vi "Chart_Formula_Manual_Fill.vi"(8 "error in (no error)":errorcluster, 10 "Max Voltage":dbl, 11 "Min Voltage":dbl) -> ()   [LabVIEW 2020]
uses:
  Global 1.vi
panel:
  out "Chosen Max Voltage":dbl
  out "Chosen Min Voltage":dbl
  out "Dummy Array":dbl[](array[numeric])
  out "size(s)":i32
  out "Output Array":dbl[](array[numeric])
  out "error out":errorcluster
  in  "Confirm Filled-up Test Voltages  ?":bool
  in  "Manual Fill In":dbl[](array[numeric])
  # "NOTE ON THE CHOSEN MIN & MAX VOLTAGE :"
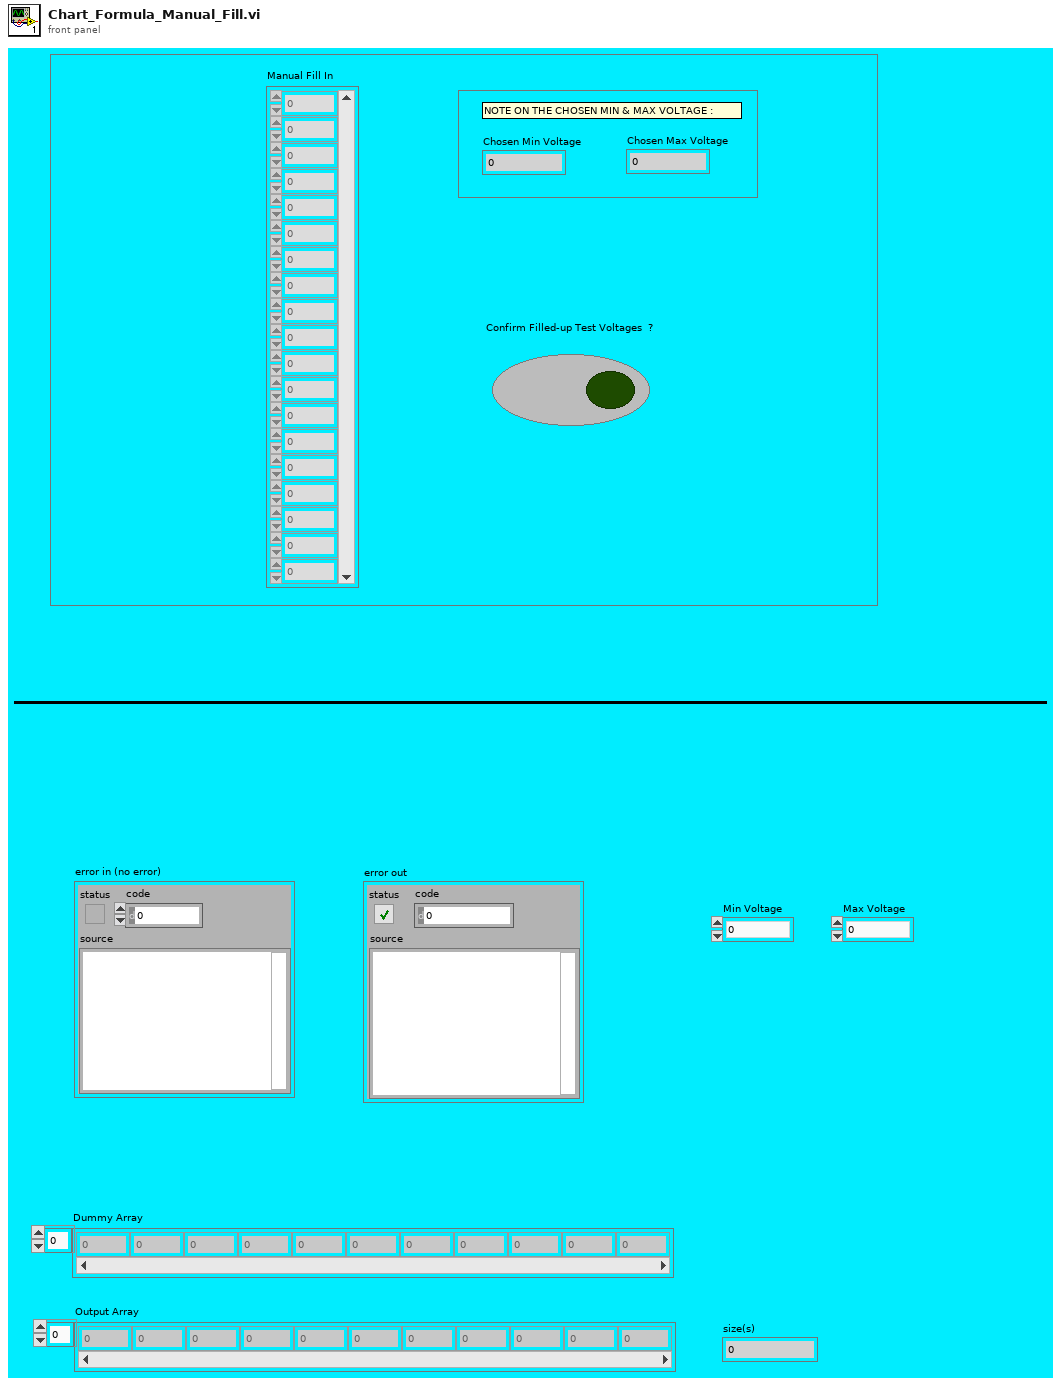
[diagram p1: front panel]
types:
  T1 = enum32{"Invalid", "Standard", "Closed", "Hidden", "Minimized", "Maximized"}
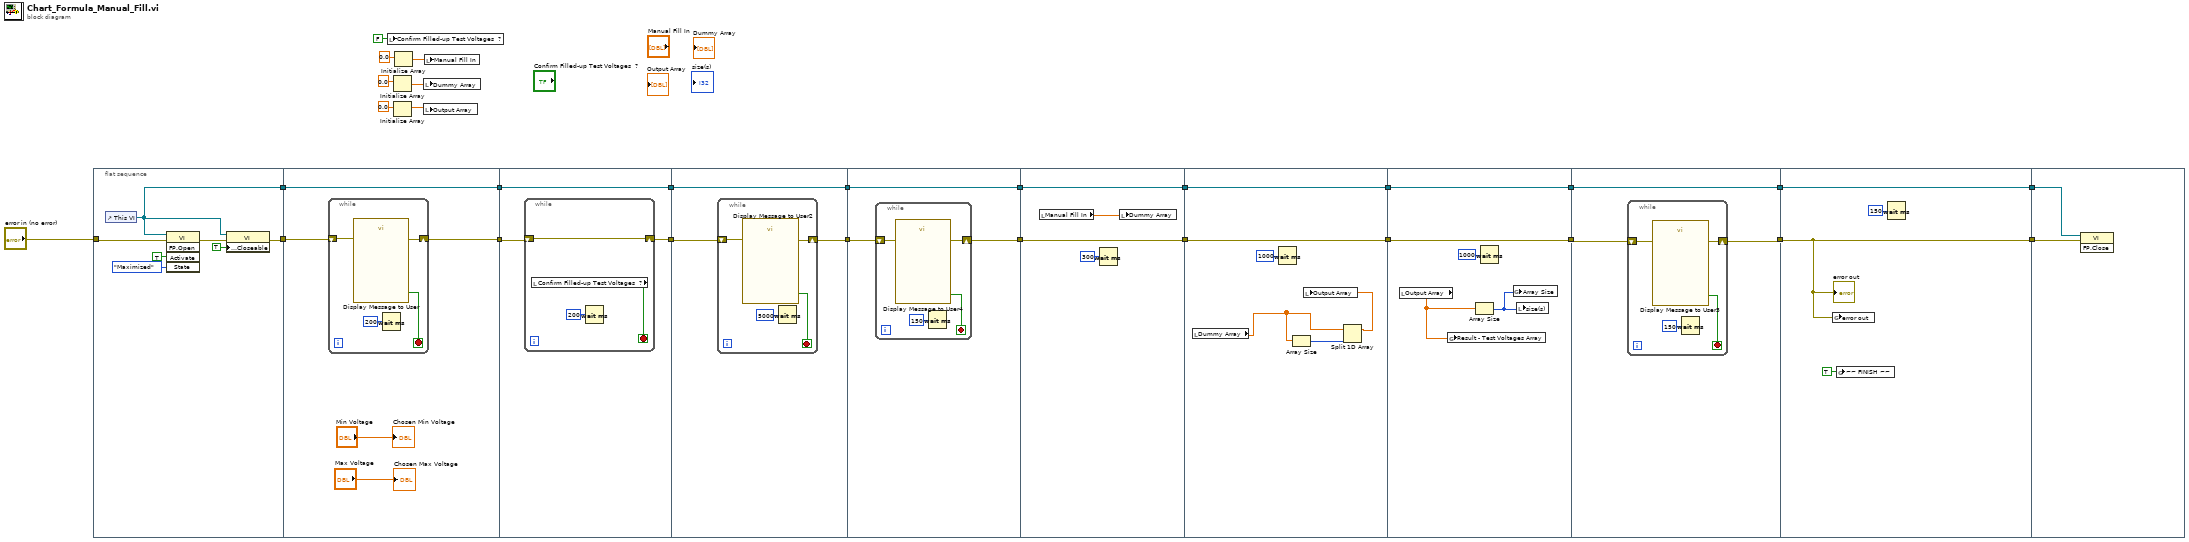
[diagram p0: block diagram]
diagram:
  n1 = flat-sequence {
    tunnel: "error in (no error)" -> [w33]
    tunnel: [w30] -> w23
    tunnel: [w29] -> w19
    tunnel: [w39] -> w25
    tunnel: w23 -> [w40]
    tunnel: [w38] -> w20
    tunnel: w19 -> [w38]
    tunnel: w25 -> [w47]
    tunnel: [w46] -> w22
    tunnel: [w45] -> w21
    tunnel: w20 -> [w45]
    tunnel: w22 -> [w53]
    tunnel: [w52] -> w6
    tunnel: w21 -> [w51]
    tunnel: [w51] -> w4
    tunnel: w6 -> [w59]
    tunnel: [w58] -> w5
    tunnel: w4 -> [w60]
    tunnel: [w60] -> w3
    tunnel: w5 -> [w68]
    tunnel: [w68] -> w18
    tunnel: [w67] -> w17
    tunnel: w3 -> [w67]
    tunnel: w18 -> [w74]
    tunnel: [w74] -> w12
    tunnel: w17 -> [w73]
    tunnel: [w73] -> w11
    tunnel: w12 -> [w79]
    tunnel: [w79] -> w10
    tunnel: w11 -> [w78]
    tunnel: [w78] -> w8
    tunnel: w10 -> [w81]
    tunnel: [w80] -> w9
    tunnel: w8 -> [w82]
    tunnel: [w82] -> w7
    tunnel: w9 -> [w88]
    tunnel: w7 -> [w89]
    tunnel: [w89] -> w2
    tunnel: [w88] -> w1
    tunnel: w2 -> [w92]
    tunnel: w1 -> [w91]
    frame #0 {
      n2 = control-ref of="This VI"() -> (w29:refnum<vi>)
      n3 = invoke class="VI" method="FP.Open"(reference=w29, error in=w33, "Activate"=TRUE ("Activate?"), "State"=T1."Maximized") -> (error out=w31:errorcluster)  [unwired: 1 in, 4 out]
      n4 = property class="VI"(reference=w29, error in=w31, "Front Panel.Closeable"=TRUE ("Front Panel Window:Closeable")) -> (error out=w30:errorcluster)  [unwired: 1 out]
    }
    frame #1 {
      n5 = while {
        shift-right: [w43] -> w39
        shift-left: w40 -> [w44]
        stop <- w41 stop-if-true
        n6 = call "Display Message to User"("error in (no error)"=w44) -> ("error out"=w43:errorcluster, "OK"=w41:bool)  [unwired: 9 in]
        n7 = Wait (ms)(milliseconds to wait=u32 200) -> ()  [unwired: 1 out]
      }
      "Chosen Min Voltage" <- "Min Voltage"
      "Chosen Max Voltage" <- "Max Voltage"
    }
    frame #2 {
      n8 = while {
        shift-right: [w49] -> w46
        shift-left: w47 -> [w49]
        stop <- w48 stop-if-true
        n9 = local read "Confirm Filled-up Test Voltages  ?"() -> (w48:bool)
        n10 = Wait (ms)(milliseconds to wait=u32 200) -> ()  [unwired: 1 out]
      }
    }
    frame #3 {
      n11 = while {
        shift-right: [w56] -> w52
        shift-left: w53 -> [w57]
        stop <- w54 stop-if-true
        n12 = call "Display Message to User2"("error in (no error)"=w57) -> ("error out"=w56:errorcluster, "YES"=w54:bool)  [unwired: 9 in]
        n13 = Wait (ms)(milliseconds to wait=u32 5000) -> ()  [unwired: 1 out]
      }
    }
    frame #4 {
      n14 = while {
        shift-right: [w63] -> w58
        shift-left: w59 -> [w64]
        stop <- w62 stop-if-true
        n15 = call "Display Message to User4"("error in (no error)"=w64) -> ("error out"=w63:errorcluster, "OK"=w62:bool)  [unwired: 9 in]
        n16 = Wait (ms)(milliseconds to wait=u32 150) -> ()  [unwired: 1 out]
      }
    }
    frame #5 {
      n17 = local read "Manual Fill In"() -> (w66:dbl[])
      n18 = Wait (ms)(milliseconds to wait=u32 300) -> ()  [unwired: 1 out]
      n19 = local write "Dummy Array"(w66) -> ()
    }
    frame #6 {
      n20 = local read "Dummy Array"() -> (w70:dbl[])
      n21 = Wait (ms)(milliseconds to wait=u32 1000) -> ()  [unwired: 1 out]
      n22 = Array Size(array=w70) -> (size(s)=w69:i32)
      n23 = Split 1D Array(array=w70, index=w69) -> (first subarray=w71:dbl[])  [unwired: 1 out]
      n24 = local write "Output Array"(w71) -> ()
    }
    frame #7 {
      n25 = local read "Output Array"() -> (w76:dbl[])
      n26 = global write "Global 1.vi" "Result - Test Voltages Array"(w76) -> ()
      n27 = Array Size(array=w76) -> (size(s)=w77:i32)
      n28 = Wait (ms)(milliseconds to wait=u32 1000) -> ()  [unwired: 1 out]
      n29 = global write "Global 1.vi" "Array Size"(w77) -> ()
      n30 = local write "size(s)"(w77) -> ()
    }
    frame #8 {
      n31 = while {
        shift-right: [w85] -> w80
        shift-left: w81 -> [w86]
        stop <- w83 stop-if-true
        n32 = call "Display Message to User3"("error in (no error)"=w86) -> ("error out"=w85:errorcluster, "OK"=w83:bool)  [unwired: 9 in]
        n33 = Wait (ms)(milliseconds to wait=u32 150) -> ()  [unwired: 1 out]
      }
    }
    frame #9 {
      n34 = global write "Global 1.vi" "error out"(w88) -> ()
      n35 = global write "Global 1.vi" "~~ FINISH ~~"(TRUE ("~~ FINISH ~~")) -> ()
      n36 = Wait (ms)(milliseconds to wait=u32 150) -> ()  [unwired: 1 out]
      "error out" <- w88
    }
    frame #10 {
      n37 = invoke class="VI" method="FP.Close"(reference=w92, error in=w91) -> ()  [unwired: 1 in, 3 out]
    }
  }
  n38 = local write "Confirm Filled-up Test Voltages  ?"(FALSE ("Confirm Filled-up Test Voltages  ?")) -> ()
  n39 = Initialize Array(0.0 ("element")) -> (w14:dbl[])  [unwired: 1 in]
  n40 = Initialize Array(0.0 ("element")) -> (w13:dbl[])  [unwired: 1 in]
  n41 = Initialize Array(0.0 ("element")) -> (w28:dbl[])  [unwired: 1 in]
  n42 = local write "Dummy Array"(w14) -> ()
  n43 = local write "Output Array"(w13) -> ()
  n44 = local write "Manual Fill In"(w28) -> ()
